vi "GetFileVersion (ActiveX).vi"(8 "error in (no error)":errorcluster, 11 "Filespec":path=path "C:/Windows/notepad.exe") -> (0 "error out":errorcluster, 1 "Version array":i32[](array[numeric]), 2 "No build version":string, 3 "Full version":string)   [LabVIEW 2017]
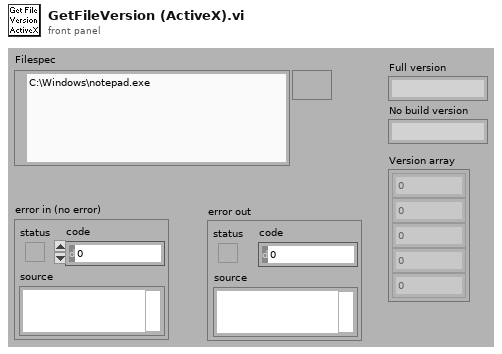
[diagram p1: front panel]
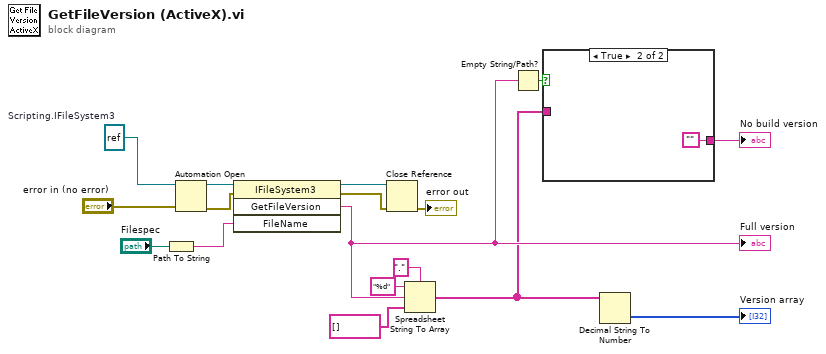
[diagram p0: block diagram]
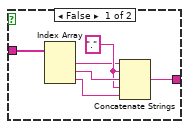
[diagram p2: hidden frame]
diagram:
  w17 = refnum<k7> refnum  # Scripting.IFileSystem3
  n1 = Path To String(path="Filespec") -> (string=w11:string)
  n2 = Automation Open(error in (no error)="error in (no error)", Automation Refnum=w17) -> (Automation Refnum=w16:refnum<k7>, error out=w15:errorcluster)  [unwired: 2 out]
  n3 = invoke class="IFileSystem3" method="GetFileVersion"(reference=w16, error in=w15, "FileName"=w11) -> (reference out=w14:refnum<k7>, error out=w13:errorcluster, "GetFileVersion"=w6:string)  [unwired: 1 in, 1 out]
  "Full version" <- w6
  n4 = Close Reference(reference=w14, error in (no error)=w13) -> (error out=→"error out":errorcluster)
  n5 = Spreadsheet String To Array(delimiter (Tab)=".", format string="%d", spreadsheet string=w6, array type (2D Dbl)=string[] []) -> (array=w4:string[])
  n6 = Empty String/Path?(string/path=w6) -> (empty?=w7:bool)
  n7 = case shown="True" w7 {
    tunnel: [w20 ""] -> w5
    tunnel: w4 -> [w19 _]
    frame False {
      w21 = "." ("delimiter (Tab)")
      n8 = Index Array(array=w19) -> (element #1=w18:string, element #2=w22:string, element #3=w23:string)  [unwired: 3 in]
      n9 = Concatenate Strings(w18, w21, w22, w21, w23) -> (w20:string)
    }
    frame True {
    }
  }
  "No build version" <- w5
  n10 = Decimal String To Number(string=w4) -> (number=→"Version array":i32[])  [unwired: 3 out]
